vi "add_to_current_aberration.vi"(11 "Zernike Coefficients":dbl[](array[numeric])) -> ()   [LabVIEW 2010]
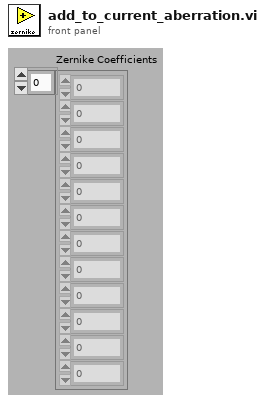
[diagram p1: front panel]
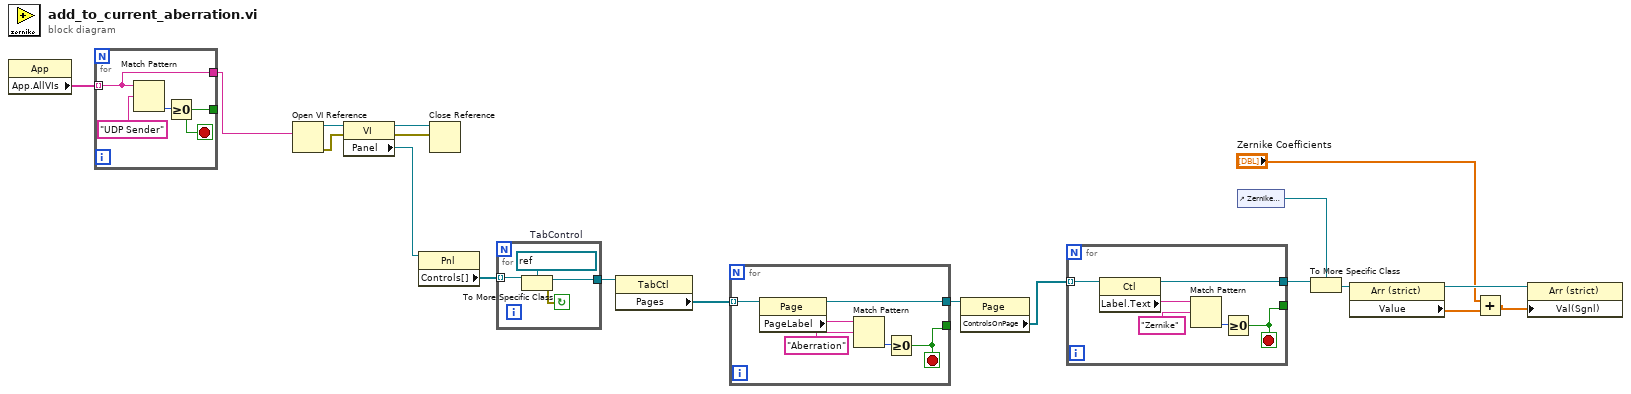
[diagram p0: block diagram]
diagram:
  n1 = property class="App"() -> ("App.AllVIs"=w19:string[])  [unwired: 2 in, 2 out]
  n2 = for {
    tunnel: w19 -> [w20] mode=indexing
    tunnel: [w21] -> _
    tunnel: [w20] -> w18
    stop <- w21 stop-if-true
    n3 = Match Pattern(string=w20, regular expression="UDP Sender") -> (offset past match=w22:i32)  [unwired: 1 in, 3 out]
    n4 = Greater Or Equal To 0?(x=w22) -> (x >= 0?=w21:bool)
  }
  n5 = Open VI Reference(vi path=w18) -> (vi reference=w17:refnum<vi>, error out=w16:errorcluster)  [unwired: 5 in]
  n6 = property class="VI"(reference=w17, error in=w16) -> (reference out=w15:refnum<vi>, error out=w14:errorcluster, "Panel"=w13:refnum<vi>)
  n7 = property class="Pnl"(reference=w13) -> ("Controls[]"=w9:refnum<vi>[])  [unwired: 1 in, 2 out]
  n8 = Close Reference(reference=w15, error in (no error)=w14) -> ()  [unwired: 1 out]
  n9 = for {
    tunnel: w9 -> [w27] mode=indexing
    tunnel: [w26] -> w8
    stop <- w25 continue-if-true
    w24 = refnum<vi> refnum  # TabControl
    n10 = To More Specific Class(target class=w24, reference=w27) -> (specific class reference=w26:refnum<vi>, error out=w25:errorcluster)  [unwired: 1 in]
  }
  n11 = property class="TabCtl"(reference=w8) -> ("Pages"=w7:refnum<vi>[])  [unwired: 1 in, 2 out]
  n12 = for {
    tunnel: w7 -> [w33] mode=indexing
    tunnel: [w31] -> _
    tunnel: [w29] -> w6
    stop <- w31 stop-if-true
    n13 = property class="Page"(reference=w33) -> (reference out=w29:refnum<vi>, "PageLabel"=w28:string)  [unwired: 1 in, 1 out]
    n14 = Match Pattern(string=w28, regular expression="Aberration") -> (offset past match=w32:i32)  [unwired: 1 in, 3 out]
    n15 = Greater Or Equal To 0?(x=w32) -> (x >= 0?=w31:bool)
  }
  n16 = property class="Page"(reference=w6) -> ("ControlsOnPage"=w5:refnum<vi>[])  [unwired: 1 in, 2 out]
  n17 = for {
    tunnel: w5 -> [w39] mode=indexing
    tunnel: [w37] -> _
    tunnel: [w35] -> w12
    stop <- w37 stop-if-true
    n18 = property class="Ctl"(reference=w39) -> (reference out=w35:refnum<vi>, "Label.Text"=w34:string)  [unwired: 1 in, 1 out]
    n19 = Match Pattern(string=w34, regular expression="Zernike") -> (offset past match=w38:i32)  [unwired: 1 in, 3 out]
    n20 = Greater Or Equal To 0?(x=w38) -> (x >= 0?=w37:bool)
  }
  n21 = control-ref of="Zernike Coefficients"() -> (w11:refnum<vi>)
  n22 = To More Specific Class(target class=w11, reference=w12) -> (specific class reference=w10:refnum<vi>)  [unwired: 1 in, 1 out]
  n23 = property class="Arr (strict)"(reference=w10) -> (reference out=w4:refnum<vi>, "Value"=w3:dbl[])  [unwired: 1 in, 1 out]
  n24 = Add(x="Zernike Coefficients", y=w3) -> (x+y=w1:dbl[])
  n25 = property class="Arr (strict)"(reference=w4, "Val(Sgnl)"=w1) -> ()  [unwired: 1 in, 2 out]
